vi "Task Unavailable Error.vi"(10 "Error/Warning (T: Error)":bool=TRUE) -> (0 "error out":errorcluster)   [LabVIEW 2017, in "Futures.lvlib" / "Task.lvclass"]
doc: "The task unavailable error/warning."
uses:
  Task.lvclass
  <vilib>/Utility/error.llb/Error Cluster From Error Code.vi
  <vilib>/ErrorRing/Error Ring.xnode
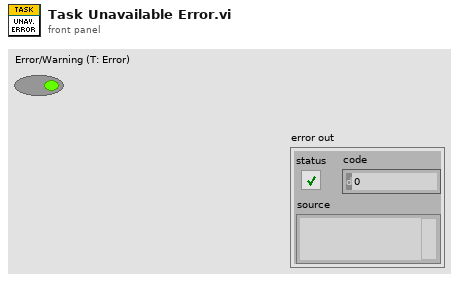
[diagram p1: front panel]
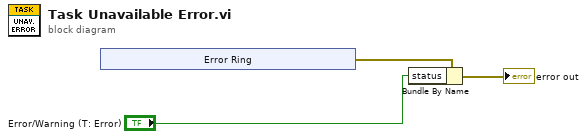
[diagram p0: block diagram]
diagram:
  n1 = xnode "Error Ring"() -> ("error out"=w3:errorcluster)
  n2 = Bundle By Name(cluster=w3, "status"="Error/Warning (T: Error)") -> (→"error out":errorcluster)
